vi "config.vi"(0 "连接ID":refnum<k5>, 1 "x":dbl, 2 "y":dbl, 3 "z":dbl, 4 "item":string(combo)="home") -> (5 "连接ID输出":refnum<k5>)   [LabVIEW 2017]
uses:
  <vilib>/LVH/i3 JSON/JSON Generation/Add Object Parameter Files/Add Object Parameter - Numeric.vi
  <vilib>/LVH/i3 JSON/i3-json.lvlib
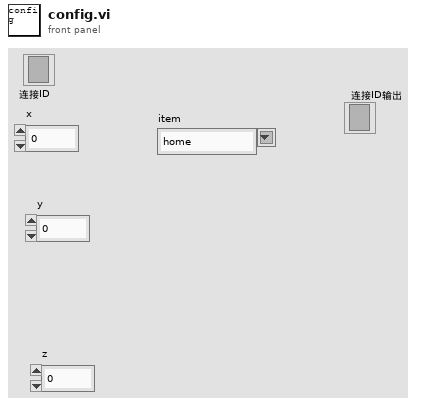
[diagram p1: front panel]
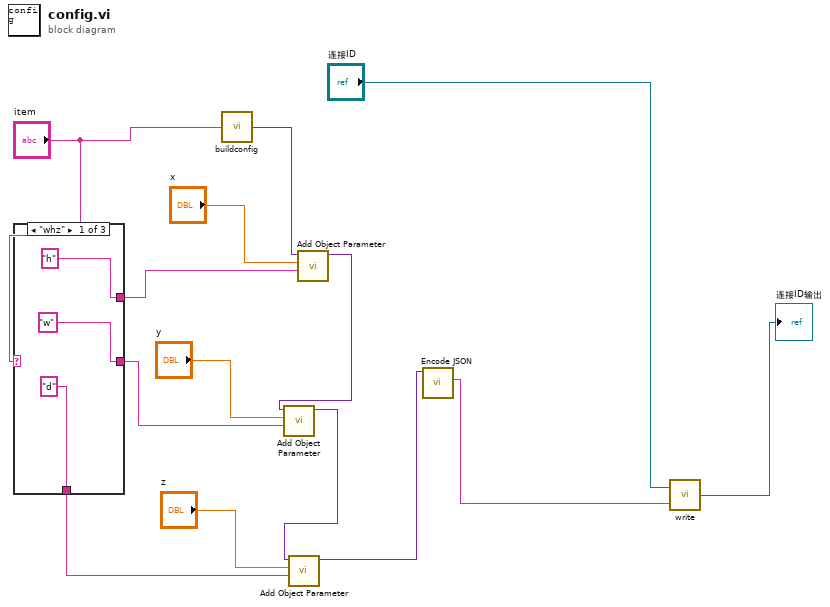
[diagram p0: block diagram]
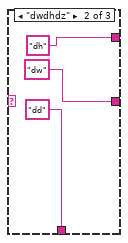
[diagram p2: hidden frame]
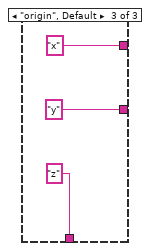
[diagram p3: hidden frame]
diagram:
  n1 = case shown="\"whz\"" "item" {
    tunnel: ["h" ("Name") "dh" ("Name") "x" ("Name")] -> w3
    tunnel: ["w" ("Name") "dw" ("Name") "y" ("Name")] -> w2
    tunnel: ["d" ("Name") "dd" ("Name") "z" ("Name")] -> w1
    frame "whz" {
    }
    frame "dwdhdz" {
    }
    frame "origin", Default {
    }
  }
  n2 = call "buildconfig.vi"("String"="item") -> ("JSON Tree out (JSON Object)"=w9:variant)
  n3 = call-poly <vilib>:"Add Object Parameter.vi"("Name"=w3, "Numeric"="x", "JSON Tree in (JSON Object)"=w9) -> ("JSON Tree out (JSON Object)"=w11:variant)  [unwired: 7 in, 1 out]
  n4 = call-poly <vilib>:"Add Object Parameter.vi"("Name"=w2, "Numeric"="y", "JSON Tree in (JSON Object)"=w11) -> ("JSON Tree out (JSON Object)"=w10:variant)  [unwired: 7 in, 1 out]
  n5 = call-poly <vilib>:"Add Object Parameter.vi"("Name"=w1, "Numeric"="z", "JSON Tree in (JSON Object)"=w10) -> ("JSON Tree out (JSON Object)"=w7:variant)  [unwired: 7 in, 1 out]
  n6 = call <vilib>:"Encode JSON.vi"("JSON Tree"=w7) -> ("String"=w6:string)  [unwired: 5 in, 1 out]
  n7 = call "write.vi"("数据输入"=w6, "连接ID"="连接ID") -> ("连接ID输出"=→"连接ID输出":refnum<k5>)
